vi "Asylum_ReadValue.vi"(8 "error in (no error)":errorcluster, 10 "Value":string, 11 "Application":refnum<k7>) -> (0 "error out":errorcluster, 2 "Value":dbl, 3 "Application":refnum<k7>)   [LabVIEW 2016]
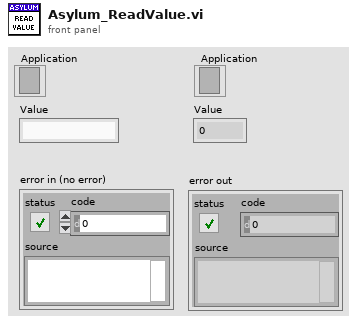
[diagram p1: front panel]
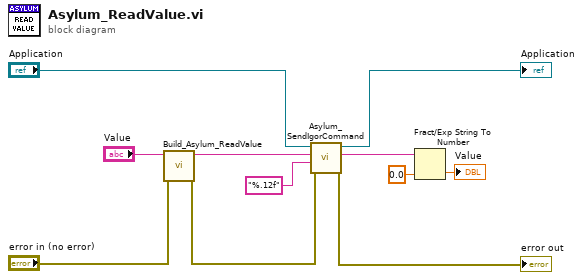
[diagram p0: block diagram]
diagram:
  n1 = call "Build_Asylum_ReadValue.vi"("error in (no error)"="error in (no error)", "Value"="Value") -> ("error out"=w1:errorcluster, "String"=w9:string)  [unwired: 8 in]
  n2 = call "Asylum_SendIgorCommand.vi"("error in (no error)"=w1, "Format"="%.12f" ("Expected output Format"), "command"=w9, "Application"="Application") -> ("error out"=→"error out":errorcluster, "results"=w4:string, "Application"=→"Application":refnum<k7>)  [unwired: 4 in, 1 out]
  n3 = Fract/Exp String To Number(string=w4, default (0 dbl)=0.0 ("default (0 DBL)")) -> (number=→"Value":dbl)  [unwired: 3 out]
